vi "create_file_path.vi"(1 "Old Temperature":dbl[](array[numeric]), 2 "Output Power (dBm)":dbl, 3 "Frequency (Hz)":dbl, 4 "Folder":path) -> (0 "file path":path)   [LabVIEW 2017]
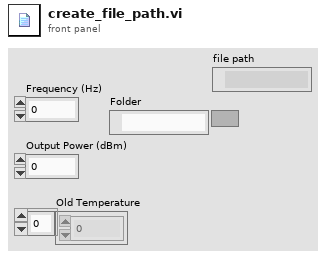
[diagram p1: front panel]
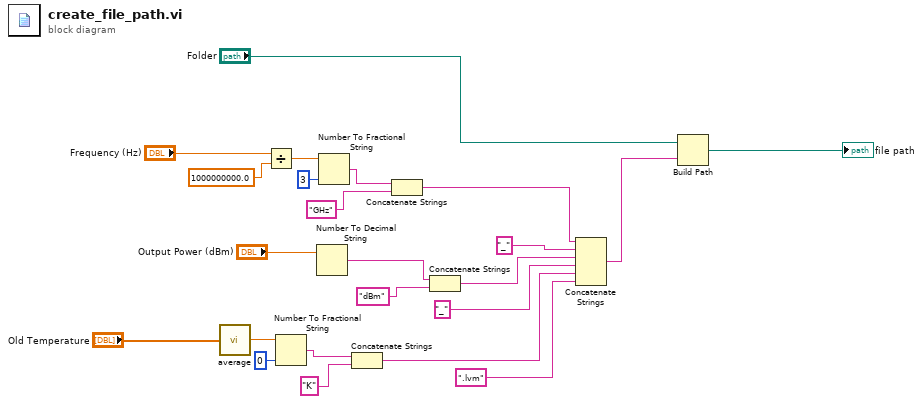
[diagram p0: block diagram]
diagram:
  n1 = call "average.vi"("Array"="Old Temperature") -> ("Average"=w14:dbl)
  n2 = Divide(x="Frequency (Hz)", y=1000000000.0) -> (x/y=w20:dbl)
  n3 = Number To Fractional String(number=w14, precision (6)=i16 0) -> (F-format string=w12:string)  [unwired: 2 in]
  n4 = Number To Decimal String(number="Output Power (dBm)") -> (decimal integer string=w8:string)  [unwired: 1 in]
  n5 = Number To Fractional String(number=w20, precision (6)=i16 3) -> (F-format string=w10:string)  [unwired: 2 in]
  n6 = Concatenate Strings(w12, "K" ("string")) -> (w2:string)
  n7 = Concatenate Strings(w10, "GHz" ("string")) -> (w6:string)
  n8 = Concatenate Strings(w8, "dBm" ("string")) -> (w4:string)
  n9 = Concatenate Strings(w6, "_" ("string"), w4, "_" ("string"), w2, ".lvm" ("string")) -> (w17:string)
  n10 = Build Path(base path="Folder", name or relative path=w17) -> (appended path=→"file path":path)
